vi "Initialize TDMS Log File.vi"(8 "error in (no error)":errorcluster, 9 "Operation":T1, 10 "File Path":path, 11 "TDMS Log File Specification in":refnum<class "TDMS Log File Specification.lvclass">) -> (0 "error out":errorcluster, 1 "Log File out":refnum<class "Log File.lvclass">, 3 "TDMS Log File Specification out":refnum<class "TDMS Log File Specification.lvclass">)   [LabVIEW 2012, in "Waveform Data Logger Shared.lvlib" / "TDMS Log File Specification.lvclass"]
uses:
  TDMS Log File Specification.lvclass
  Engine/Classes/Logs/Log Files/Log File/Log File.lvclass
  Engine/Classes/Logs/Log Files/Log File/Operation.ctl
  Log File Specification/Log File Specification.lvclass/Log File Specification.ctl
  TDMS Log File Specification.lvclass/TDMS Log File Specification.ctl
  Engine/Classes/Logs/Log Files/TDMS Log File/TDMS Log File.lvclass
  Engine/Classes/Logs/Log Files/TDMS Log File/TDMS Log File.lvclass/TDMS Log File.ctl
  Log File Specification/Log File Specification.lvclass
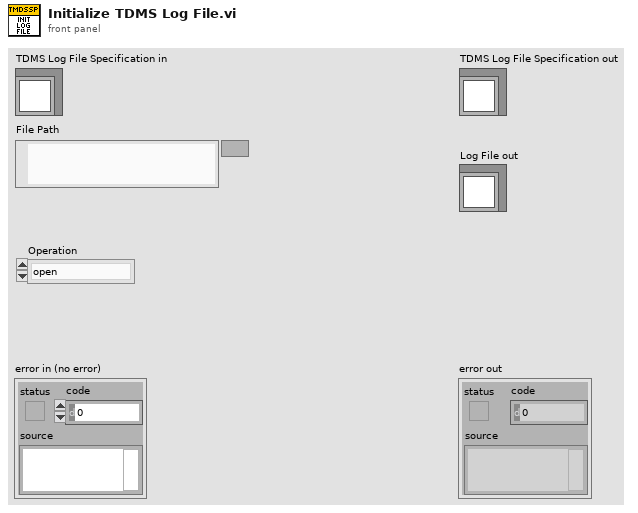
[diagram p1: front panel]
types:
  T1 = typedef "Waveform Data Logger Engine.lvlib/Log File.lvclass/Operation.ctl" = enum16{"open", "open or create", "create or replace", "create", "open (read-only)"}
  T2 = typedef "Waveform Data Logger Shared.lvlib/TDMS Log File Specification.lvclass/Channel Group Specification.ctl" = cluster{"Name":string, "Properties":T3[], "Channels":T4[]}
  T3 = typedef "Waveform Data Logger Shared.lvlib/TDMS Log File Specification.lvclass/Property Specification.ctl" = cluster{"Name":string, "Value":variant}
  T4 = typedef "Waveform Data Logger Shared.lvlib/TDMS Log File Specification.lvclass/Channel Specification.ctl" = cluster{"Name":string, "Properties":T3[]}
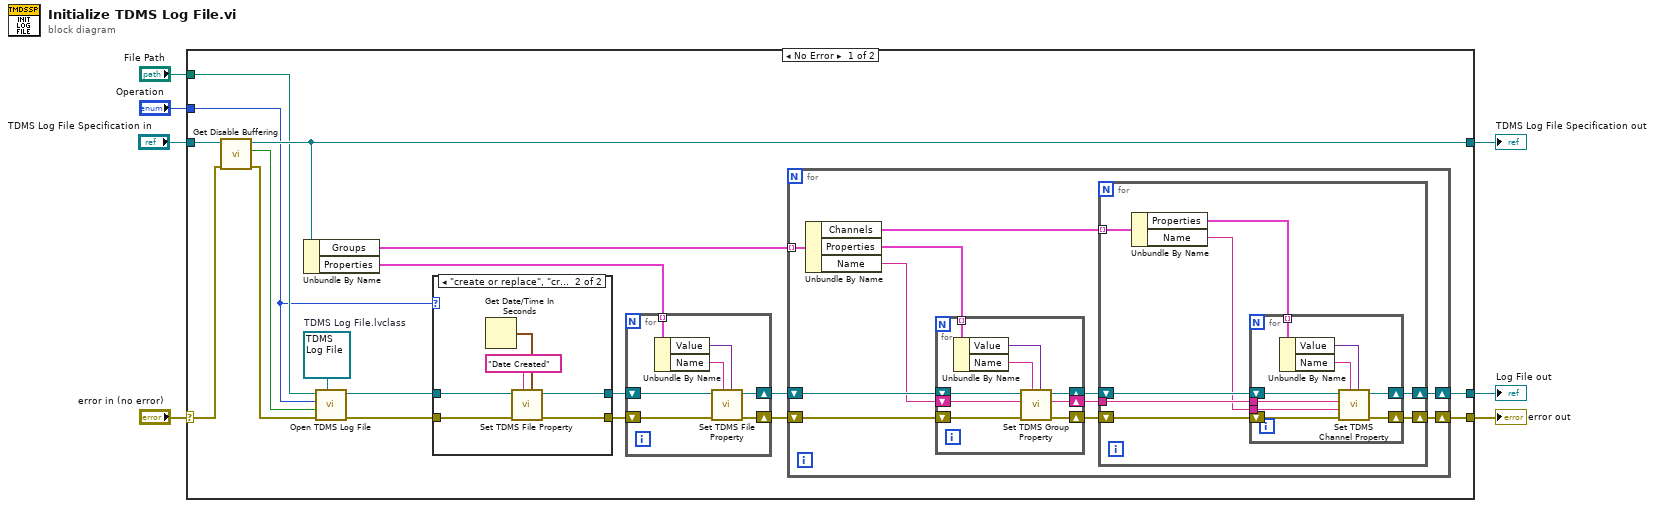
[diagram p0: block diagram]
diagram:
  n1 = case shown="No Error" "error in (no error)" {
    selector: "error in (no error)" -> [w24 w78]
    tunnel: [w17 w79] -> w6
    tunnel: "TDMS Log File Specification in" -> [w23 w79]
    tunnel: [w19 w78] -> w4
    tunnel: "File Path" -> [w16 _]
    tunnel: "Operation" -> [w8 _]
    tunnel: [w18 _] -> w1
    frame No Error {
      w15 = refnum<class "TDMS Log File.lvclass"> refnum  # TDMS Log File.lvclass
      n2 = call "Get Disable Buffering.vi"("error in (no error)"=w24, "Log File Specification in"=w23) -> ("error out"=w25:errorcluster, "Disable Buffering"=w22:bool, "Log File Specification out"=w17:refnum<class "TDMS Log File Specification.lvclass">)  [unwired: 7 in]
      n3 = Unbundle By Name(w17) -> ("Groups"=w20:T2[], "Properties"=w21:T3[])
      n4 = call "Open TDMS Log File.vi"("TDMS Log File Type"=w15, "error in (no error)"=w25, "Disable Buffering (F)"=w22, "Operation"=w8, "File Path"=w16) -> ("error out"=w11:errorcluster, "TDMS Log File out"=w12:refnum<class "TDMS Log File.lvclass">)  [unwired: 5 in]
      n5 = case shown="\"create or replace\", \"create\"" w8 {
        tunnel: w12 -> [w27 w31]
        tunnel: w11 -> [w26 w30]
        tunnel: [w27 w29] -> w10
        tunnel: [w26 w28] -> w9
        frame Default {
        }
        frame "create or replace", "create" {
          n6 = Get Date/Time In Seconds() -> (seconds since 1Jan1904=w32:timestamp)
          n7 = call "Set TDMS File Property.vi"("Property Value"=w32, "Property Name"="Date Created" ("property names"), "error in (no error)"=w30, "TDMS Log File in"=w31) -> ("error out"=w28:errorcluster, "TDMS Log File out"=w29:refnum<class "TDMS Log File.lvclass">)  [unwired: 6 in]
        }
      }
      n8 = for {
        tunnel: w21 -> [w77] mode=indexing
        shift-right: [w76] -> w14
        shift-left: w10 -> [w75]
        shift-right: [w73] -> w13
        shift-left: w9 -> [w74]
        n9 = Unbundle By Name(w77) -> ("Value"=w71:variant, "Name"=w72:string)
        n10 = call "Set TDMS File Property.vi"("Property Value"=w71, "Property Name"=w72, "error in (no error)"=w74, "TDMS Log File in"=w75) -> ("error out"=w73:errorcluster, "TDMS Log File out"=w76:refnum<class "TDMS Log File.lvclass">)  [unwired: 6 in]
      }
      n11 = for {
        shift-right: [w37] -> w18
        shift-left: w14 -> [w43]
        shift-right: [w36] -> w19
        shift-left: w13 -> [w42]
        tunnel: w20 -> [w44] mode=indexing
        n12 = Unbundle By Name(w44) -> ("Channels"=w40:T4[], "Properties"=w41:T3[], "Name"=w35:string)
        n13 = for {
          tunnel: w41 -> [w51] mode=indexing
          shift-right: [w50] -> w39
          shift-left: w43 -> [w53]
          shift-right: [w47] -> w34
          shift-left: w35 -> [w48]
          shift-right: [w49] -> w38
          shift-left: w42 -> [w52]
          n14 = Unbundle By Name(w51) -> ("Value"=w45:variant, "Name"=w46:string)
          n15 = call "Set TDMS Group Property.vi"("Property Value"=w45, "Property Name"=w46, "error in (no error)"=w52, "Group Name in"=w48, "TDMS Log File in"=w53) -> ("error out"=w49:errorcluster, "Group Name out"=w47:string, "TDMS Log File out"=w50:refnum<class "TDMS Log File.lvclass">)  [unwired: 4 in]
        }
        n16 = for {
          tunnel: w40 -> [w60] mode=indexing
          shift-right: [w55] -> w37
          shift-left: w39 -> [w59]
          shift-right: [w54] -> w36
          shift-left: w38 -> [w58]
          tunnel: w34 -> [w57]
          n17 = Unbundle By Name(w60) -> ("Properties"=w61:T3[], "Name"=w56:string)
          n18 = for {
            tunnel: w61 -> [w70] mode=indexing
            shift-right: [w65] -> w55
            shift-left: w59 -> [w69]
            shift-right: [w64] -> w54
            shift-left: w58 -> [w68]
            tunnel: w57 -> [w63]
            tunnel: w56 -> [w62]
            n19 = Unbundle By Name(w70) -> ("Value"=w67:variant, "Name"=w66:string)
            n20 = call "Set TDMS Channel Property.vi"("Property Value"=w67, "Property Name"=w66, "error in (no error)"=w68, "Channel Name in"=w62, "Group Name in"=w63, "TDMS Log File in"=w69) -> ("error out"=w64:errorcluster, "TDMS Log File out"=w65:refnum<class "TDMS Log File.lvclass">)  [unwired: 2 in, 2 out]
          }
        }
      }
    }
    frame Error {
    }
  }
  "error out" <- w4
  "TDMS Log File Specification out" <- w6
  "Log File out" <- w1
